vi "drive to destination.vi"() -> ()   [LabVIEW 2010, in "GyroDrive.lvrbt"]
uses:
  GyroDrive/GyroDrive.lvrbt
  <vilib>/Platform/TimedLoop/XDataNode/wakeup.ctl
  <vilib>/Platform/TimedLoop/XDataNode/XDNodeRunTimeDep.lvlib
  <vilib>/Platform/TimedLoop/XDataNode/nitl_modes.ctl
  <vilib>/Platform/TimedLoop/XDataNode/timing_clust.ctl
  <vilib>/Platform/TimedLoop/XDataNode/XDataNode.xnode
  <vilib>/NXT/Dual Mode Library/Sensors/Sonar_cm.vi
  <vilib>/NXT/Block Support/NXT_InputPort.ctl
panel:
  out "End":i32
  out "Waveform Chart 2":i16(graph)
  out "Waveform Chart":i16(graph)
  in  "Destination In":dbl
  out "Mode":string
  out "Timmer Count":dbl
  in  "stop":bool
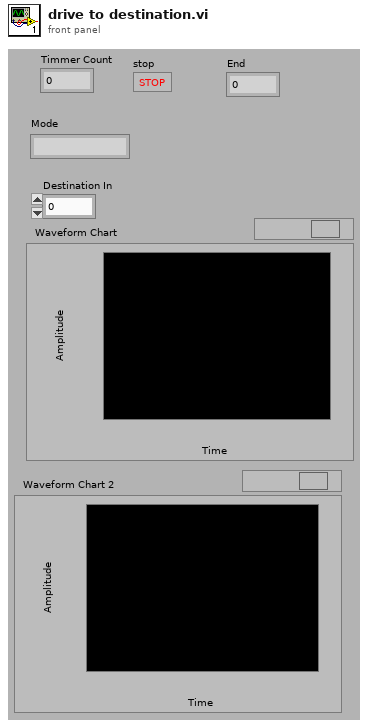
[diagram p1: front panel]
types:
  T1 = typedef "XDNodeRunTimeDep.lvlib/timing_clust.ctl" = cluster{"Expected End [f-1]":u64, "Actual End [f-1]":u64, "Finished Late? [f-1]":bool, "Expected End [i-1]":u64, "Actual End [i-1]":u64, "Finished Late? [i-1]":bool, "Expected Start [i]":u64, "Actual Start [i]":u64, "Expected Start [f]":u64, "Actual Start [f]":u64, "Source Name":string, "Structure Name":string, "Period":i64, "Deadline":i64, "Offset":i64, "Start":i64, "Priority":i32, "Timeout":i32, "Mode":T2, "Wakeup Reason":T3, "Error":errorcluster, "Source Type":string, "Secondary Source Type":string, "Global End Time":u64, "Global Start Time":u64, "Frame Duration":u64, "Iteration Duration":u64, "Assigned CPU":i32, "I/O Scan Engine Mode":u32}
  T2 = typedef "XDNodeRunTimeDep.lvlib/nitl_modes.ctl" = enum32{"No Change", "Process missed periods, maintain original phase", "Discard missed periods, maintain original phase", "Process missed periods, ignore original phase", "Discard missed periods, ignore original phase"}
  T3 = typedef "XDNodeRunTimeDep.lvlib/wakeup.ctl" = enum32{"Normal", "Aborted", "Asynchronous wakeup", "Timing source error", "Timed loop error", "Timeout"}
  T4 = typedef "NXT_InputPort.ctl" = u8
  T5 = typedef "LVHSConnector.ctl" = cluster{"Hardware":string, "Flattened String":string}
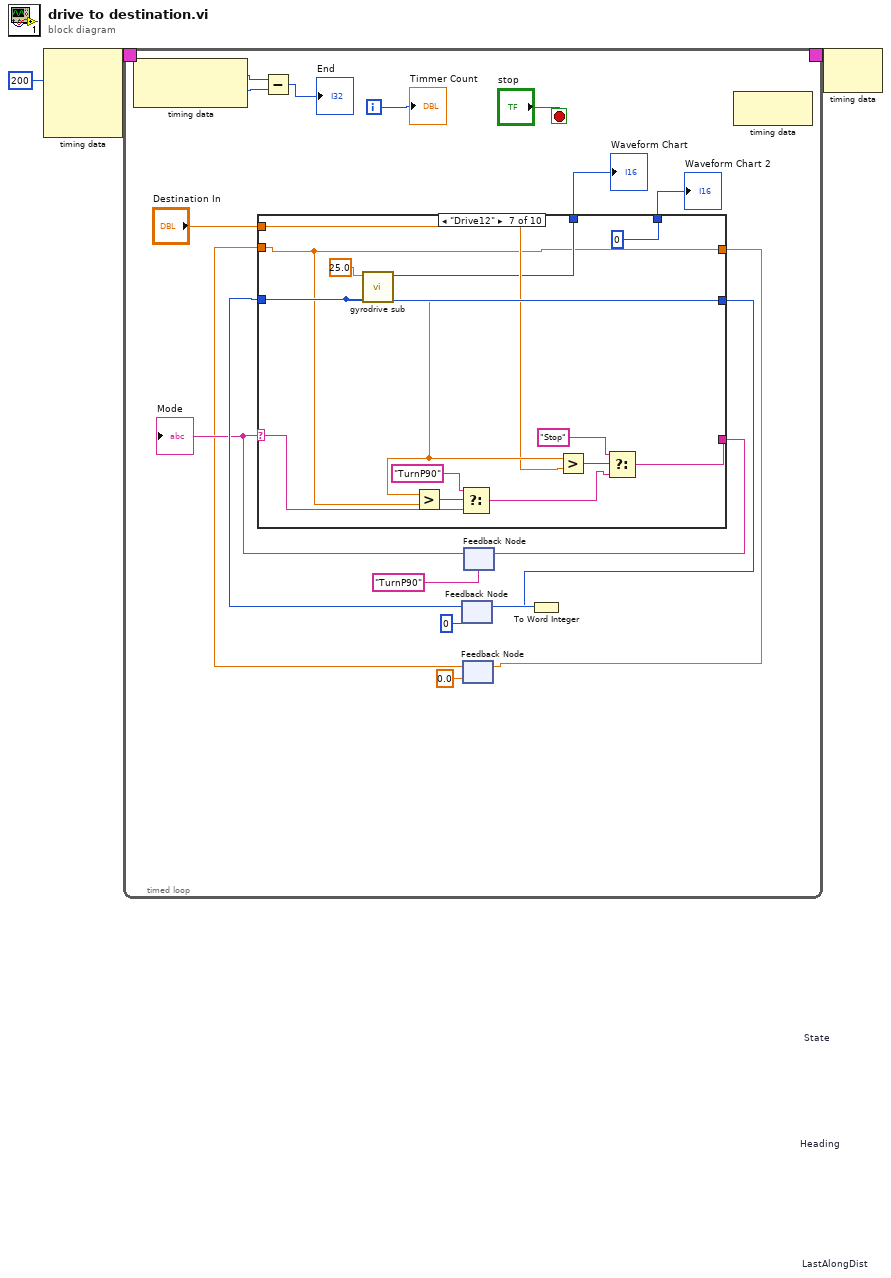
[diagram p0: block diagram]
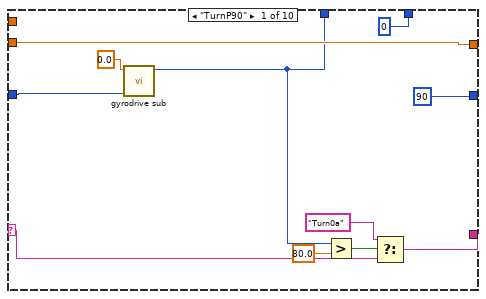
[diagram p2: hidden frame]
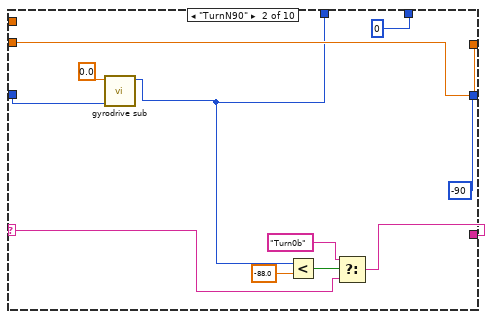
[diagram p3: hidden frame]
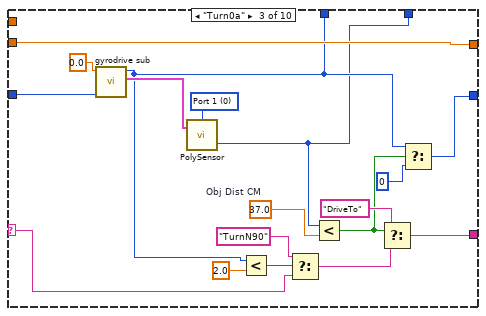
[diagram p4: hidden frame]
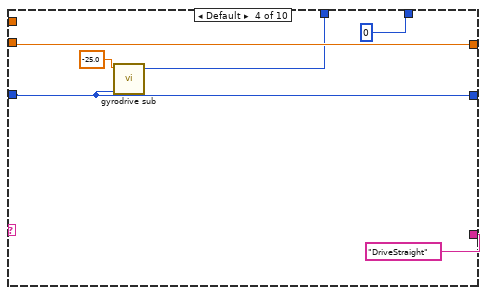
[diagram p5: hidden frame]
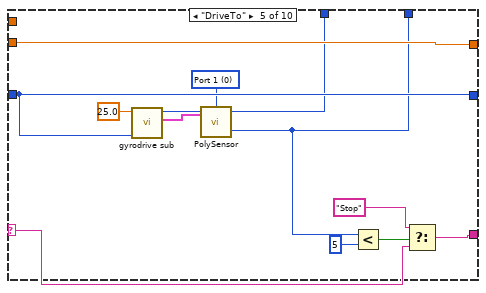
[diagram p6: hidden frame]
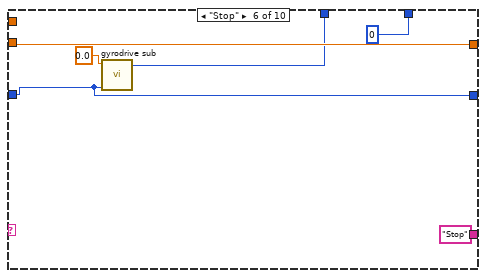
[diagram p7: hidden frame]
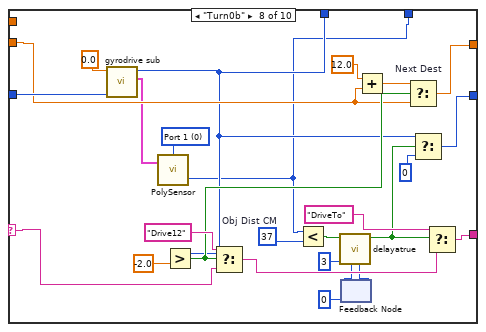
[diagram p8: hidden frame]
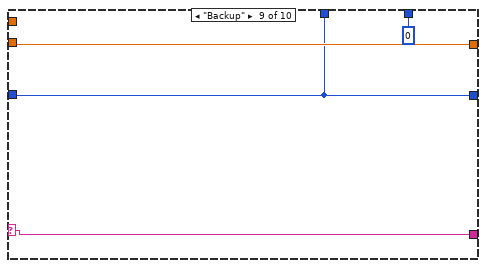
[diagram p9: hidden frame]
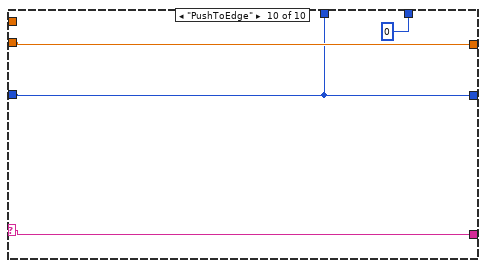
[diagram p10: hidden frame]
diagram:
  n1 = node-c288(i64 200 ("Period")) -> (w3:T1)  [unwired: 3 in]
  n2 = timed-loop {
    timing: w3 -> [_]
    timing-out: [_] -> w2
    i -> [w21]
    stop <- "stop" stop-if-true
    n3 = node-c288() -> (w5:i64, w4:i64)  [unwired: 1 in]
    n4 = Subtract(x=w5, y=w4) -> (x-y=→"End":i64)
    n5 = feedback #1 "Heading"(i16 0) -> (w19:i16)
    n6 = feedback #2 "LastAlongDist"(0.0 ("Along Dist In")) -> (w10:dbl)
    n7 = feedback #3 "State"("TurnP90") -> (w13:string)
    "Mode" <- w13
    n8 = case shown="\"Drive12\"" w13 {
      selector: w13 -> [w25 w36 w56 _ w73 _ w93 w121 w128 w132]
      tunnel: w19 -> [w30 w42 w60 w64 w71 w84 w98 w122 w127 w131]
      tunnel: [i16 90 i16 -90 w50 w64 w71 w84 w98 w107 w127 w131] -> w16
      tunnel: [w26 w37 w51 "DriveStraight" w75 "Stop" w96 w113 w128 w132] -> w14
      tunnel: [w24 w35 w55 w65 w72 w82 w87 w118 w129 w133] -> w12
      tunnel: w10 -> [w24 w35 w55 w65 w72 w82 w87 w116 w129 w133]
      tunnel: "Destination In" -> [_ _ _ _ _ _ w89 _ _ _]
      tunnel: [w23 w34 w46 w63 w69 w81 w88 w108 w127 w131] -> w8
      tunnel: [i16 0 ("Distance (cm)") i16 0 ("Distance (cm)") w44 i16 0 ("Distance (cm)") w68 i16 0 ("Distance (cm)") i16 0 ("Distance (cm)") w106 i16 0 ("Distance (cm)") i16 0 ("Distance (cm)")] -> w7
      frame "TurnP90" {
        n9 = call "gyrodrive sub.vi"("Dir Cmd"=w30, "Spd Cmd"=0.0) -> ("Hdg CKW Deg"=w23:i16)  [unwired: 6 in, 3 out]
        n10 = Greater?(x=w23, y=80.0) -> (0:w29:bool)
        n11 = Select(t="Turn0a", s=w29, f=w25) -> (s? t:f=w26:string)
      }
      frame "TurnN90" {
        n12 = call "gyrodrive sub.vi"("Dir Cmd"=w42, "Spd Cmd"=0.0) -> ("Hdg CKW Deg"=w34:i16)  [unwired: 6 in, 3 out]
        n13 = Less?(x=w34, y=-88.0) -> (x < y?=w40:bool)
        n14 = Select(t="Turn0b", s=w40, f=w36) -> (s? t:f=w37:string)
      }
      frame "Turn0a" {
        w47 = T4 0 items=["Port 1", "Port 2", "Port 3", "Port 4"] ("Port (Port 4)")
        w54 = 37.0  # Obj Dist CM
        n15 = call "gyrodrive sub.vi"("Dir Cmd"=w60, "Spd Cmd"=0.0) -> ("NXT"=w48:T5, "Hdg CKW Deg"=w46:i16)  [unwired: 6 in, 2 out]
        n16 = call-poly <vilib>:"PolySensor.vi"("NXT"=w48, "Port (Port 4)"=w47) -> ("Distance (cm)"=w44:i16)  [unwired: 1 in, 1 out]
        n17 = Less?(x=w46, y=2.0) -> (x < y?=w59:bool)
        n18 = Select(t="TurnN90", s=w59, f=w56) -> (s? t:f=w52:string)
        n19 = Less?(x=w44, y=w54) -> (x < y?=w45:bool)
        n20 = Select(t="DriveTo", s=w45, f=w52) -> (s? t:f=w51:string)
        n21 = Select(t=w46, s=w45, f=0) -> (s? t:f=w50:i32)
      }
      frame Default {
        n22 = call "gyrodrive sub.vi"("Dir Cmd"=w64, "Spd Cmd"=-25.0) -> ("Hdg CKW Deg"=w63:i16)  [unwired: 6 in, 3 out]
      }
      frame "DriveTo" {
        w70 = T4 0 items=["Port 1", "Port 2", "Port 3", "Port 4"] ("Port (Port 4)")
        n23 = call "gyrodrive sub.vi"("Dir Cmd"=w71, "Spd Cmd"=25.0) -> ("NXT"=w78:T5, "Hdg CKW Deg"=w69:i16)  [unwired: 6 in, 2 out]
        n24 = call-poly <vilib>:"PolySensor.vi"("NXT"=w78, "Port (Port 4)"=w70) -> ("Distance (cm)"=w68:i16)  [unwired: 1 in, 1 out]
        n25 = Less?(x=w68, y=i16 5) -> (x < y?=w74:bool)
        n26 = Select(t="Stop", s=w74, f=w73) -> (s? t:f=w75:string)
      }
      frame "Stop" {
        n27 = call "gyrodrive sub.vi"("Dir Cmd"=w84, "Spd Cmd"=0.0) -> ("Hdg CKW Deg"=w81:i16)  [unwired: 6 in, 3 out]
      }
      frame "Drive12" {
        n28 = call "gyrodrive sub.vi"("Dir Cmd"=w98, "Spd Cmd"=25.0) -> ("Along Dist In"=w90:dbl, "Hdg CKW Deg"=w88:i16)  [unwired: 6 in, 2 out]
        n29 = Greater?(x=w90, y=w87) -> (0:w91:bool)
        n30 = Select(t="TurnP90", s=w91, f=w93) -> (s? t:f=w92:string)
        n31 = Greater?(x=w90, y=w89) -> (0:w97:bool)
        n32 = Select(t="Stop", s=w97, f=w92) -> (s? t:f=w96:string)
      }
      frame "Turn0b" {
        w110 = T4 0 items=["Port 1", "Port 2", "Port 3", "Port 4"] ("Port (Port 4)")
        w111 = 37  # Obj Dist CM
        n33 = call "gyrodrive sub.vi"("Dir Cmd"=w122, "Spd Cmd"=0.0) -> ("NXT"=w109:T5, "Hdg CKW Deg"=w108:i16)  [unwired: 6 in, 2 out]
        n34 = call-poly <vilib>:"PolySensor.vi"("NXT"=w109, "Port (Port 4)"=w110) -> ("Distance (cm)"=w106:i16)  [unwired: 1 in, 1 out]
        n35 = Greater?(x=w108, y=-2.0) -> (0:w120:bool)
        n36 = Select(t="Drive12", s=w120, f=w121) -> (s? t:f=w112:string)
        n37 = Less?(x=w106, y=w111) -> (x < y?=w104:bool)
        n38 = feedback #4(0) -> (w100:i32)
        n39 = call "delayatrue.vi"("Z1 In"=w100, "Delay Cycles"=3, "In"=w104) -> ("Out"=w103:bool, "Z1 Out"=w101:i32)  [unwired: 7 in]
        n40 = feedback-in #4(w101) -> ()
        n41 = Add(x=12.0 ("y"), y=w116) -> (x+y=w119:dbl)
        n42 = Select "Next Dest"(t=w119, s=w120, f=w116) -> (s? t:f=w118:dbl)
        n43 = Select(t=w108, s=w103, f=0) -> (s? t:f=w107:i32)
        n44 = Select(t="DriveTo", s=w103, f=w112) -> (s? t:f=w113:string)
      }
      frame "Backup" {
      }
      frame "PushToEdge" {
      }
    }
    "Waveform Chart" <- w8
    "Waveform Chart 2" <- w7
    n45 = feedback-in #2(w12) -> ()
    n46 = feedback-in #3(w14) -> ()
    n47 = To Word Integer(number=w16) -> (16bit integer=w18:i16)
    n48 = feedback-in #1(w18) -> ()
    n49 = node-c288() -> ()  [unwired: 1 in, 1 out]
    "Timmer Count" <- w21
  }
  n50 = node-c288(w2) -> ()  [unwired: 1 out]
